vi "Maps Manager.vi"() -> ()   [LabVIEW 2014]
uses:
  <vilib>/Utility/miscctls.llb/LVPointDoubleTypeDef.ctl
  <vilib>/Utility/config.llb/Config Data RefNum.ctl
  Gps Map Graph enum.ctl
  Gps Map Graph config.ctl
  <vilib>/Utility/config.llb/Read Key (Double).vi
  <vilib>/Utility/config.llb/Write Key (Double).vi
  <vilib>/Utility/config.llb/Write Key (Path).vi
  <vilib>/ErrorRing/Error Ring.xnode
  <vilib>/Utility/config.llb/NI_LVConfig.lvlib
  My Graphs.lvlib
panel:
  in  "Points":T1[](array[typedef]) {"X" step=1e-05 format="%#_10g"; "Y" step=1e-05 format="%#_10g"}
  in  "Remove last":bool
  in  "Exit":bool
  out "Dati punto":string[][](array[string])
  in  "Save configurations":bool
  in  "North limit":dbl
  in  "South limit":dbl
  in  "East limit":dbl
  in  "West limit":dbl
  in  "Add point":bool
  in  "Load maps":bool
  in  "Load or create configurations":bool
  out "Zoom":cluster{"X":dbl, "Y":dbl}[](graph)
  out "My map":cluster{"X":dbl, "Y":dbl}[](graph)
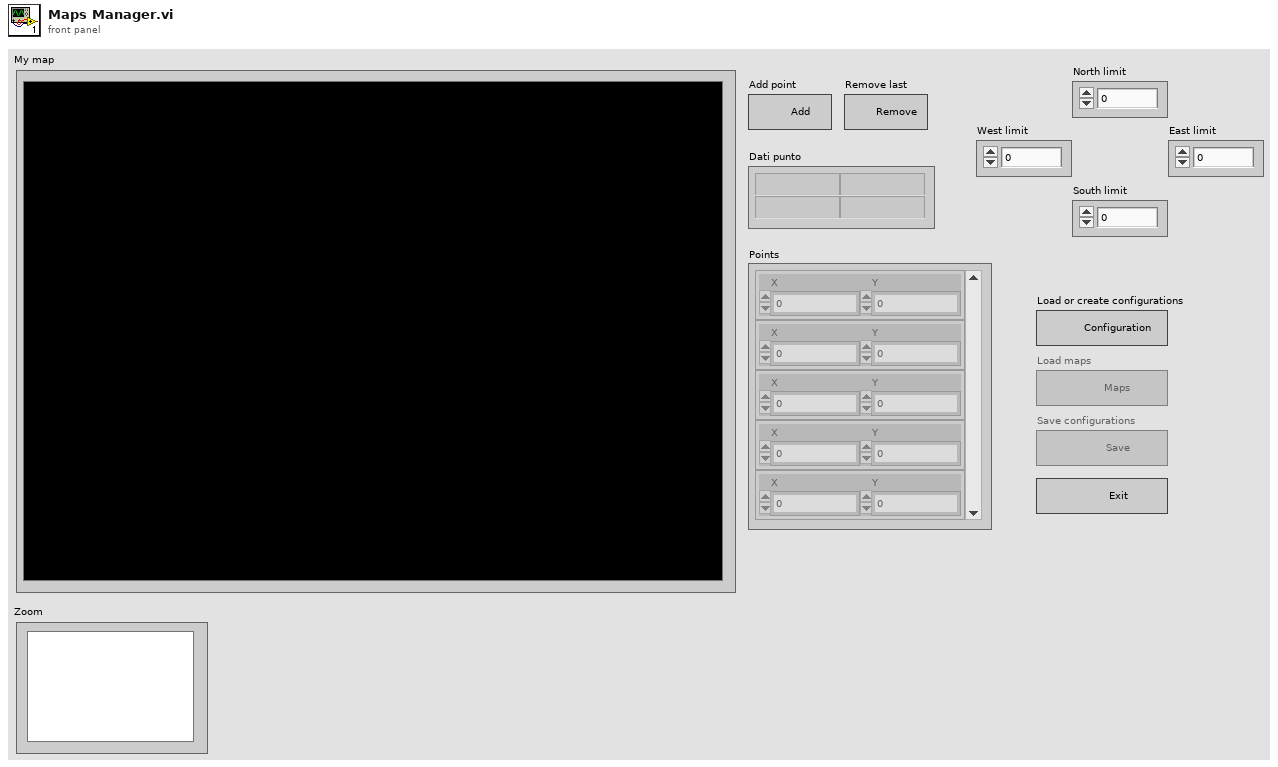
[diagram p1: front panel]
types:
  T1 = typedef "LVPointDoubleTypeDef.ctl" = cluster{"X":dbl, "Y":dbl}
  T2 = typedef "NI_LVConfig.lvlib/Config Data RefNum.ctl" = refnum<k1>
  T3 = cluster{"Config file?":bool, "Config file path":path, "Config file ref":T2, "Map files?":bool, "Big map file path":path, "Small map file path":path, "Path of points":T1[]}
  T4 = enum8{"Enabled", "Disabled", "Disabled and Grayed Out"}
  T5 = typedef "Gps Map Graph config.ctl" = cluster{"Config path":path, "Image path":path}
  T6 = typedef "My Graphs.lvlib/Gps Map Graph enum.ctl" = enum16{"Reset_ini", "Reset_txt", "SetValue"}
  T7 = typedef "imagedata.ctl" = cluster{"image type":i32, "image depth":i32, "image":u8[], "mask":u8[], "colors":u32[], "Rectangle":cluster{"left":i16, "top":i16, "right":i16, "bottom":i16}}
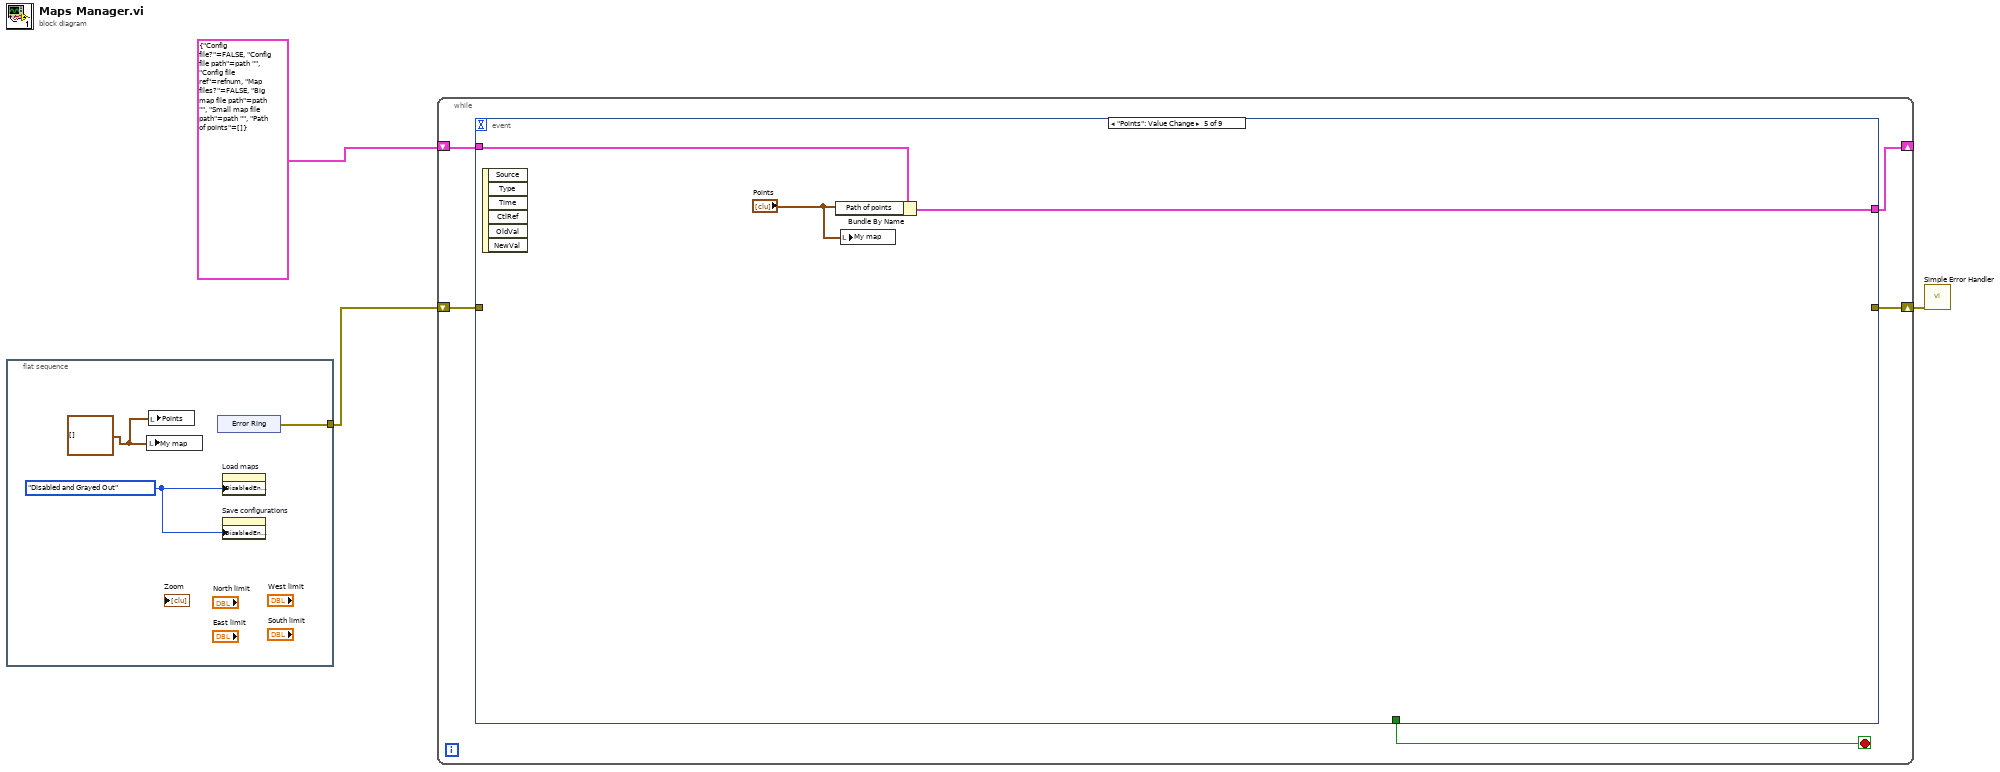
[diagram p0: block diagram]
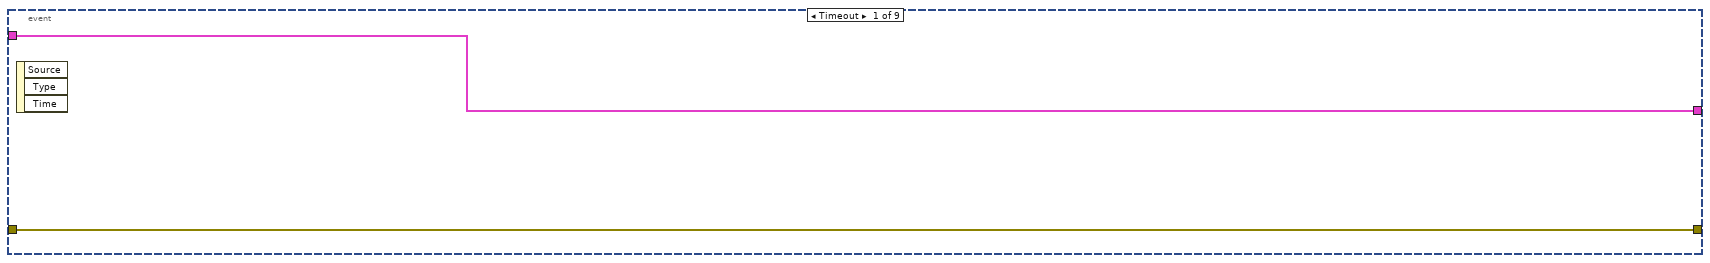
[diagram p2: hidden frame]
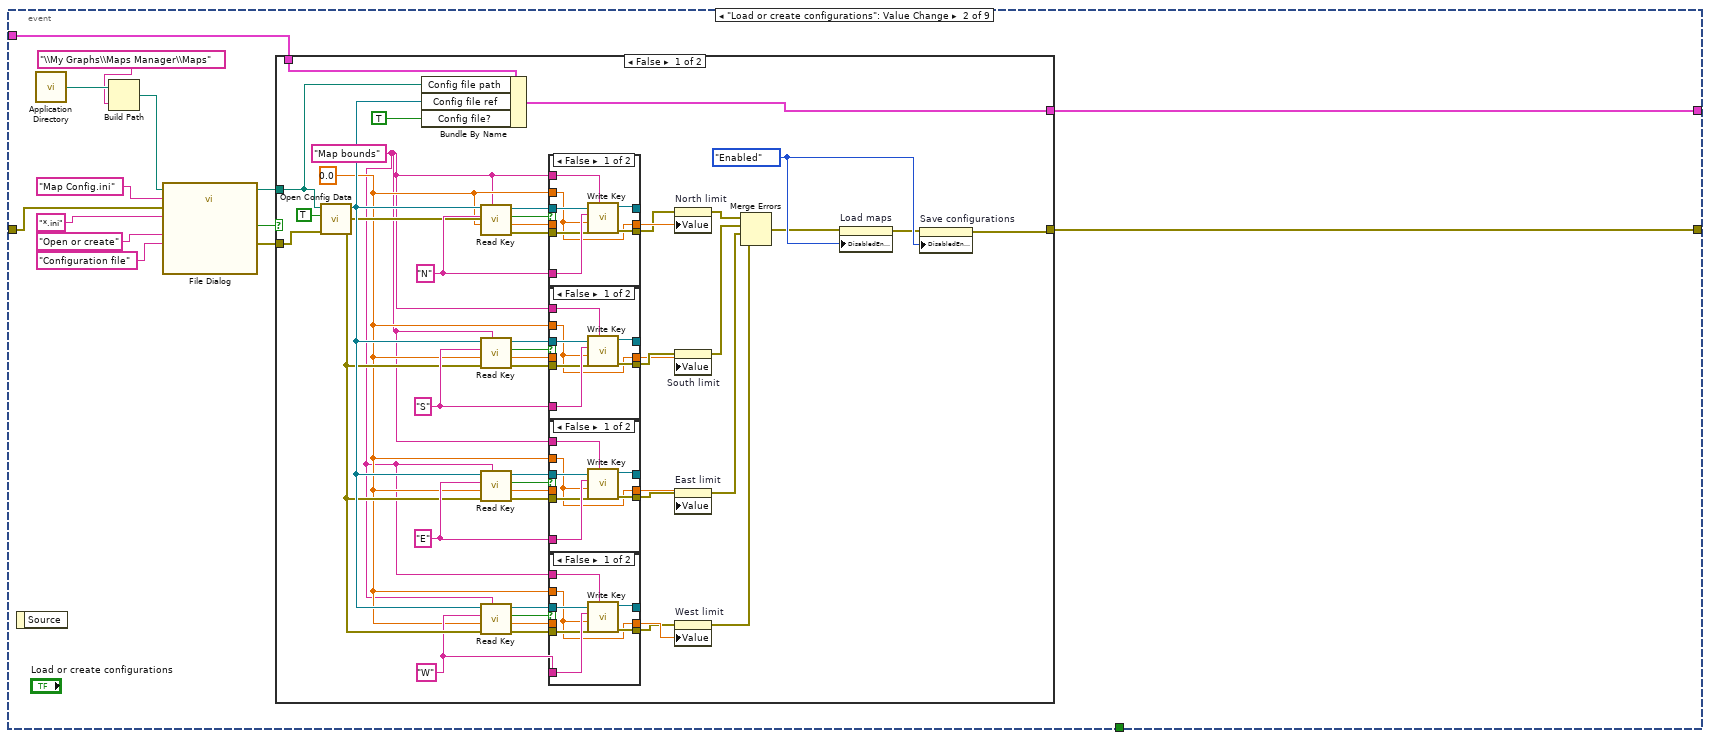
[diagram p3: hidden frame]
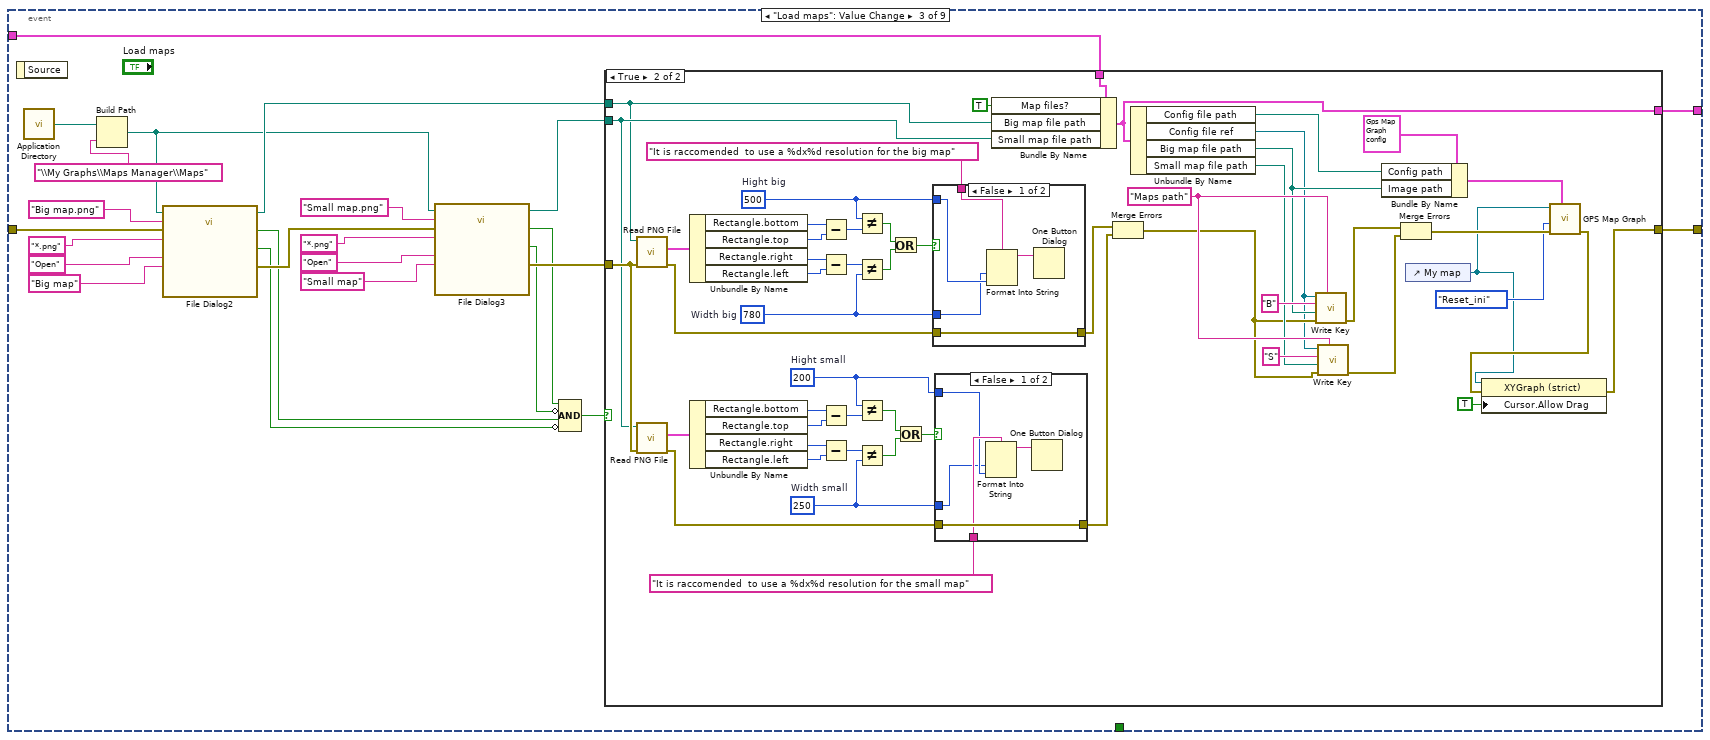
[diagram p9: hidden frame]
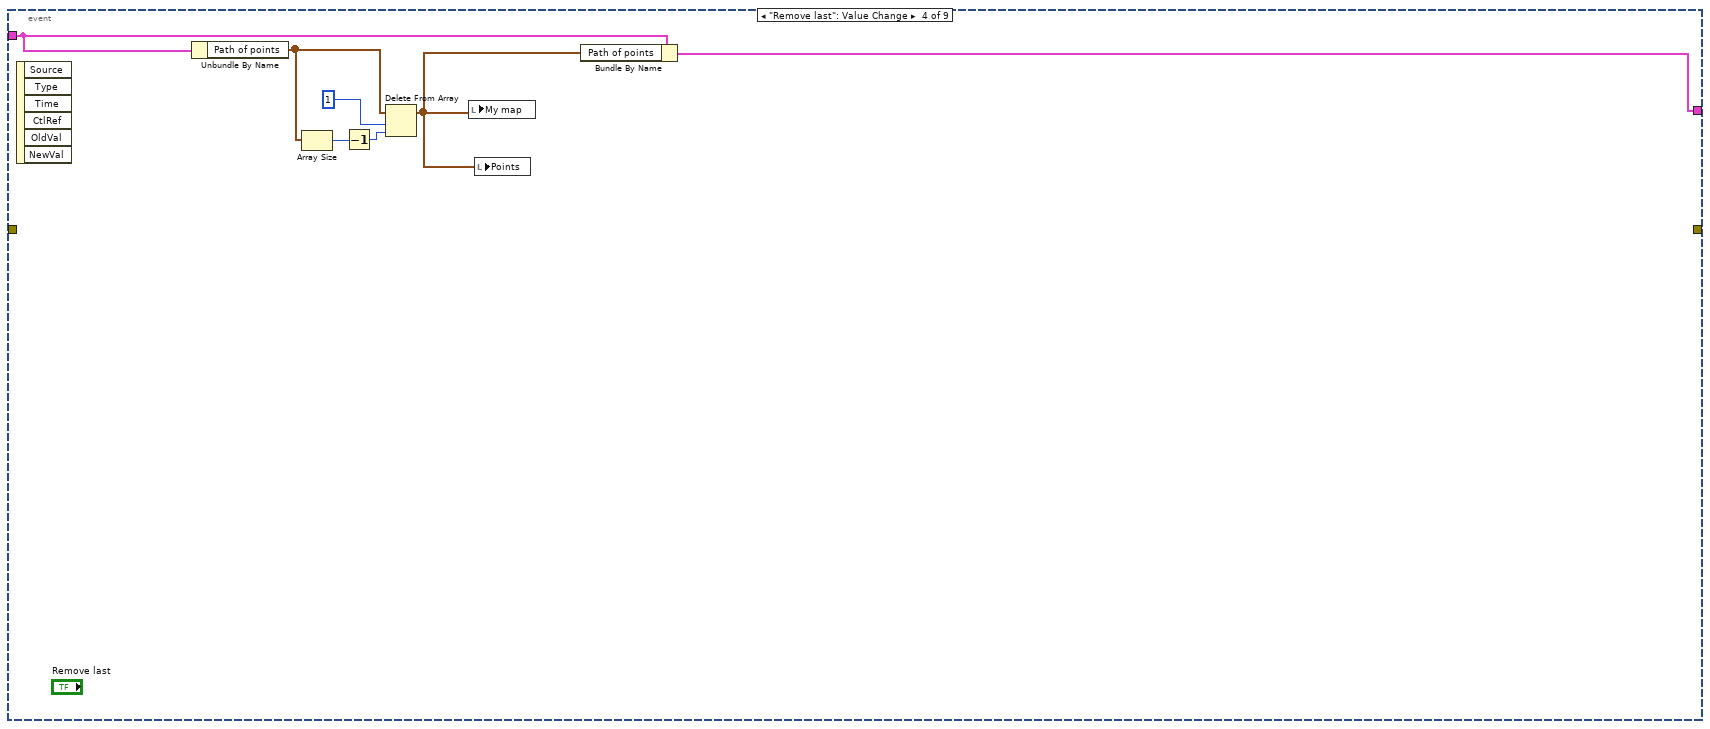
[diagram p13: hidden frame]
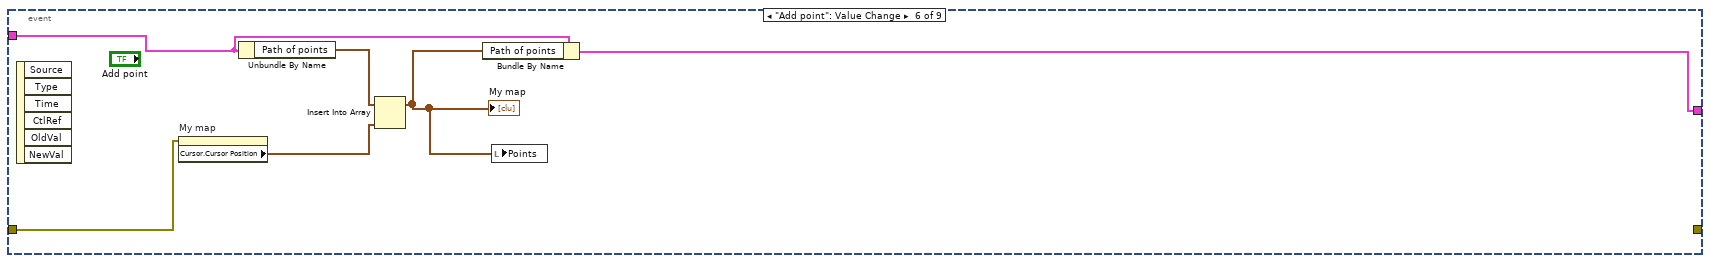
[diagram p14: hidden frame]
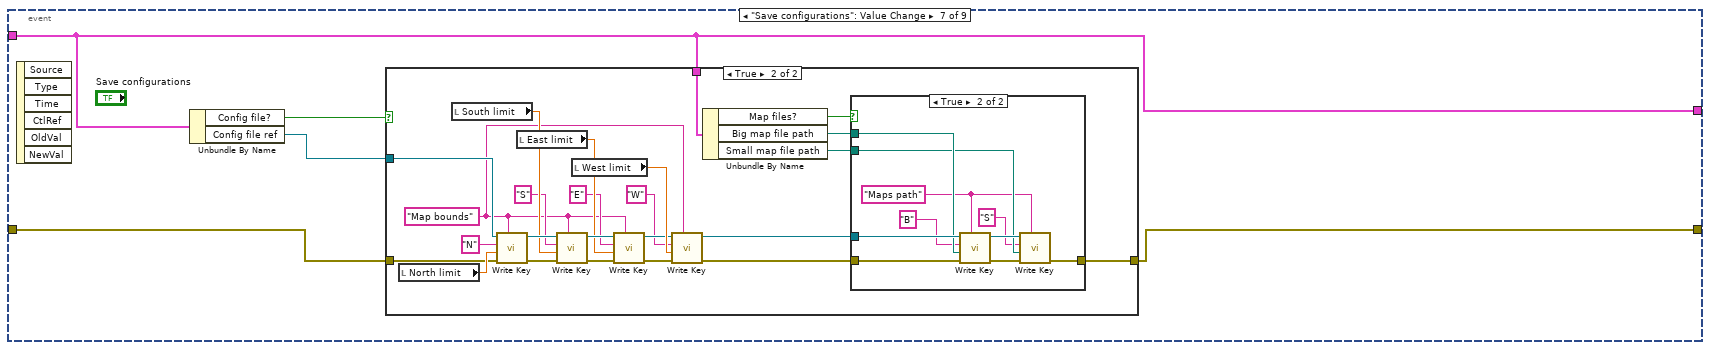
[diagram p15: hidden frame]
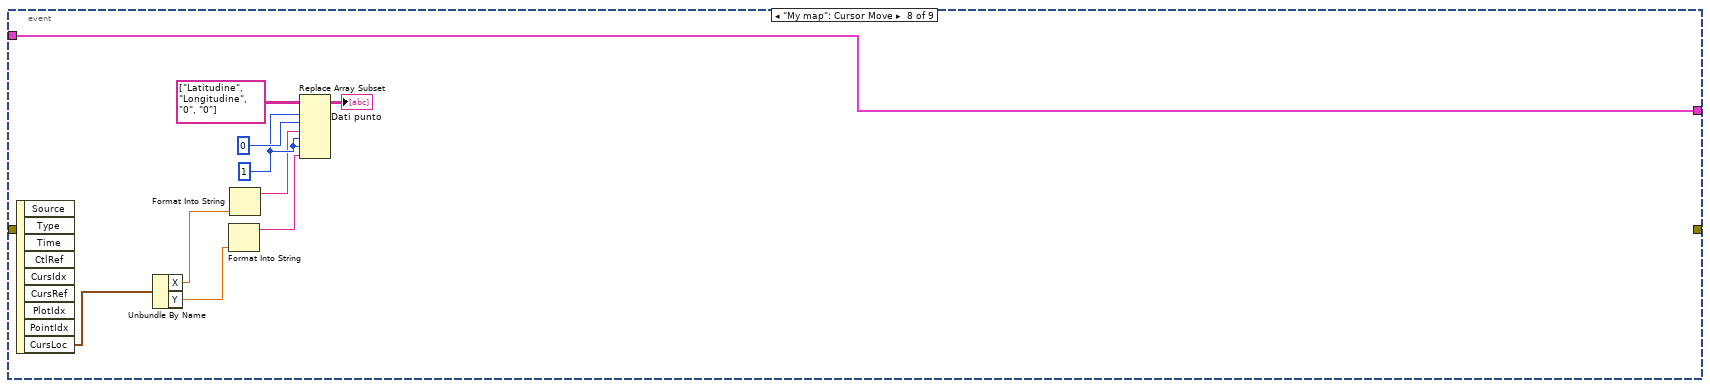
[diagram p18: hidden frame]
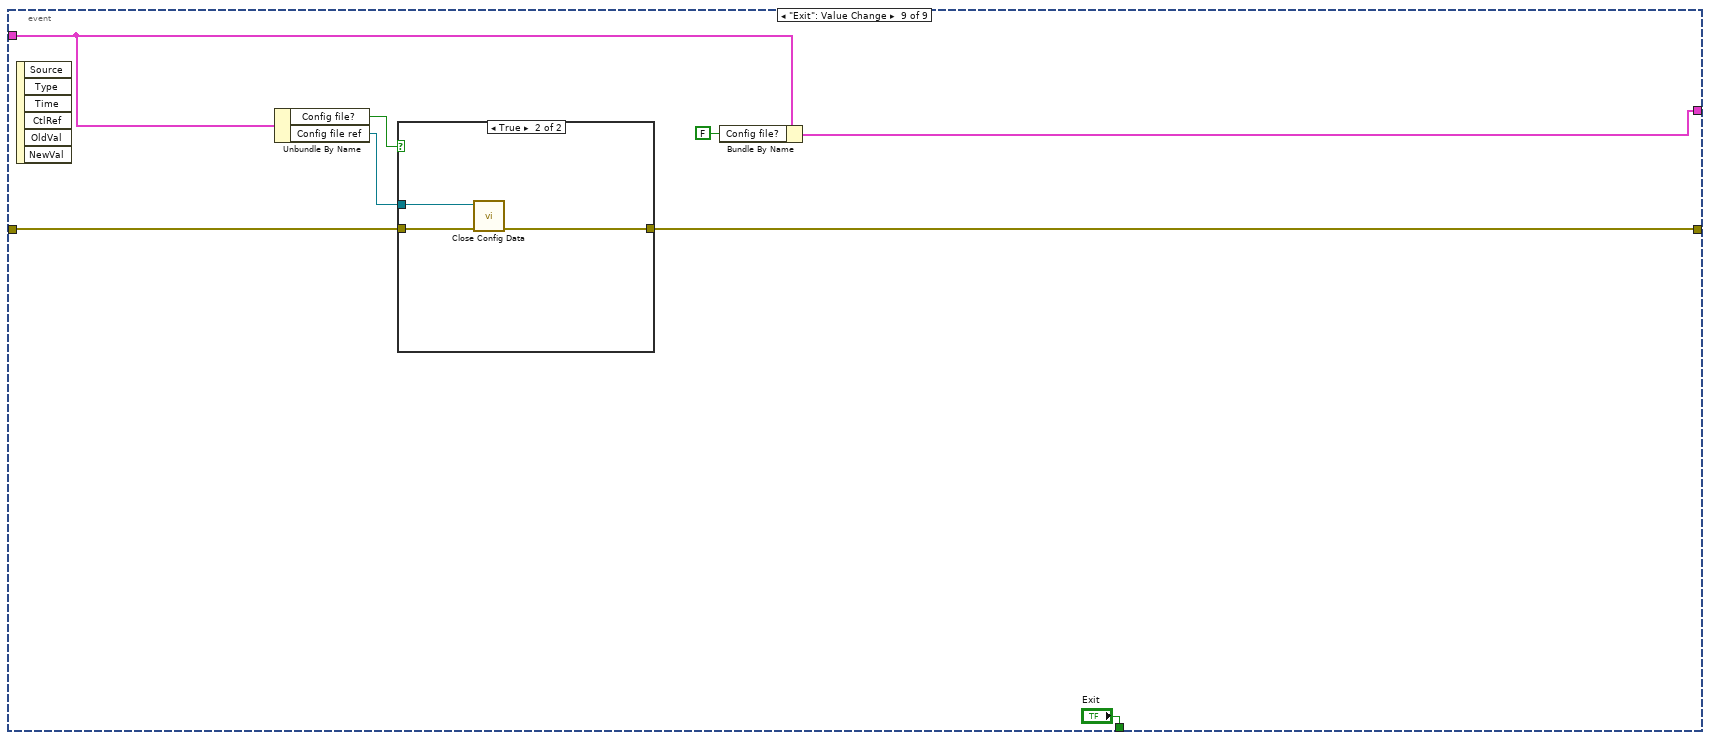
[diagram p19: hidden frame]
diagram:
  n1 = flat-sequence {
    tunnel: [w6] -> w3
    frame #0 {
      w4 = cluster{"X":i32, "Y":i32}[] [] ("My map")
      w5 = T4."Disabled and Grayed Out" ("Disabled")
      n2 = local write "My map"(w4) -> ()
      n3 = local write "Points"(w4) -> ()
      n4 = xnode "Error Ring"() -> ("error out"=w6:errorcluster)
      n5 = property on="Load maps" class="Bool"("DisabledEnum"=w5) -> ()  [unwired: 2 in, 2 out]
      n6 = property on="Save configurations" class="Bool"("DisabledEnum"=w5) -> ()  [unwired: 2 in, 2 out]
    }
  }
  n7 = while {
    shift-right: [w10] -> _
    shift-left: T3 {"Config file?"=FALSE, "Config file path"=path "", "Config file ref"=refnum, "Map files?"=FALSE, "Big map file path"=path "", "Small map file path"=path "", "Path of points"=[]} -> [w11]
    shift-right: [w9] -> w1
    shift-left: w3 -> [w12]
    stop <- w8 stop-if-true
    n8 = event shown="[4] \"Points\": Value Change" {
      selector: _ -> [_ _ _ _ _ _ _ _ _]
      dyn-events: _ -> [_ _ _ _ _ _ _ _ _]
      timeout: _ -> [_ _ _ _ _ _ _ _ _]
      tunnel: w12 -> [w13 w28 w136 _ _ w224 w227 _ w282]
      tunnel: [w13 w21 w120 _ _ _ w226 _ w281] -> w9
      tunnel: w11 -> [w14 w19 w121 w215 w218 w223 w225 w266 w278]
      tunnel: [w14 w18 w122 w214 w217 w222 w225 w266 w276] -> w10
      tunnel: [_ _ _ _ _ _ _ _ "Exit"] -> w8
      event Timeout {
        n9 = event-data() -> ()  [unwired: 1 in, 3 out]
      }
      event "Load or create configurations": Value Change {
        n10 = event-data() -> ()  [unwired: 1 in, 1 out]
        n11 = call <vilib>:"Application Directory.vi"() -> ("Application Directory"=w17:path)
        n12 = Build Path(base path=w17, name or relative path="\\My Graphs\\Maps Manager\\Maps") -> (appended path=w15:path)
        n13 = call "File Dialog"("start path"=w15, "prompt"="Configuration file", "button label"="Open or create", "default name"="Map Config.ini", "error in"=w28, "pattern (all files)"="*.ini") -> ("selected path"=w20:path, "cancelled"=w22:bool, "error out"=w23:errorcluster)  [unwired: 6 in, 1 out]
        n14 = case shown="False" w22 {
          tunnel: w23 -> [w71 w116]
          tunnel: [w30 w116] -> w21
          tunnel: w20 -> [w29 _]
          tunnel: w19 -> [w74 w115]
          tunnel: [w72 w115] -> w18
          frame False {
            w33 = T4."Enabled" ("Disabled")
            w46 = "W" ("key")
            w49 = "E" ("key")
            w48 = "S" ("key")
            w44 = "Map bounds" ("section")
            w65 = "N" ("key")
            w45 = 0.0 ("default value")
            n15 = call <vilib>:"Open Config Data.vi"("error in (no error)"=w71, "create file if necessary (T)"=TRUE, "configuration file path"=w29) -> ("error out"=w47:errorcluster, "refnum"=w50:T2)  [unwired: 6 in, 1 out]
            n16 = Bundle By Name(cluster=w74, "Config file path"=w29, "Config file ref"=w50, "Config file?"=TRUE) -> (w72:T3)
            n17 = call-poly <vilib>:"Read Key.vi"("section"=w44, "error in (no error)"=w47, "default value"=w45, "key"=w65, "refnum"=w50) -> ("error out"=w66:errorcluster, "value"=w67:dbl, "found?"=w69:bool, "refnum out"=w68:T2)  [unwired: 3 in]
            n18 = call-poly <vilib>:"Read Key.vi"("section"=w44, "error in (no error)"=w47, "default value"=w45, "key"=w48, "refnum"=w50) -> ("error out"=w59:errorcluster, "value"=w60:dbl, "found?"=w62:bool, "refnum out"=w61:T2)  [unwired: 3 in]
            n19 = call-poly <vilib>:"Read Key.vi"("section"=w44, "error in (no error)"=w47, "default value"=w45, "key"=w49, "refnum"=w50) -> ("error out"=w55:errorcluster, "value"=w56:dbl, "found?"=w58:bool, "refnum out"=w57:T2)  [unwired: 3 in]
            n20 = call-poly <vilib>:"Read Key.vi"("section"=w44, "error in (no error)"=w47, "default value"=w45, "key"=w46, "refnum"=w50) -> ("error out"=w51:errorcluster, "value"=w52:dbl, "found?"=w54:bool, "refnum out"=w53:T2)  [unwired: 3 in]
            n21 = case shown="False" w69 {
              tunnel: w68 -> [w111 w112]
              tunnel: w67 -> [_ w113]
              tunnel: w66 -> [w108 w114]
              tunnel: w65 -> [w109 _]
              tunnel: w44 -> [w110 _]
              tunnel: w45 -> [w106 _]
              tunnel: [w107 w114] -> w63
              tunnel: [w106 w113] -> w64
              tunnel: [w105 w112] -> _
              frame False {
                n22 = call-poly <vilib>:"Write Key.vi"("section"=w110, "error in (no error)"=w108, "value"=w106, "key"=w109, "refnum"=w111) -> ("error out"=w107:errorcluster, "refnum out"=w105:T2)  [unwired: 4 in, 1 out]
              }
              frame True {
              }
            }
            n23 = case shown="False" w62 {
              tunnel: w61 -> [w101 w102]
              tunnel: w60 -> [_ w103]
              tunnel: w59 -> [w98 w104]
              tunnel: w48 -> [w99 _]
              tunnel: w44 -> [w100 _]
              tunnel: w45 -> [w96 _]
              tunnel: [w97 w104] -> w43
              tunnel: [w96 w103] -> w38
              tunnel: [w95 w102] -> _
              frame False {
                n24 = call-poly <vilib>:"Write Key.vi"("section"=w100, "error in (no error)"=w98, "value"=w96, "key"=w99, "refnum"=w101) -> ("error out"=w97:errorcluster, "refnum out"=w95:T2)  [unwired: 4 in, 1 out]
              }
              frame True {
              }
            }
            n25 = case shown="False" w58 {
              tunnel: w57 -> [w91 w92]
              tunnel: w56 -> [_ w93]
              tunnel: w55 -> [w88 w94]
              tunnel: w49 -> [w89 _]
              tunnel: w44 -> [w90 _]
              tunnel: w45 -> [w86 _]
              tunnel: [w87 w94] -> w39
              tunnel: [w86 w93] -> w40
              tunnel: [w85 w92] -> _
              frame False {
                n26 = call-poly <vilib>:"Write Key.vi"("section"=w90, "error in (no error)"=w88, "value"=w86, "key"=w89, "refnum"=w91) -> ("error out"=w87:errorcluster, "refnum out"=w85:T2)  [unwired: 4 in, 1 out]
              }
              frame True {
              }
            }
            n27 = case shown="False" w54 {
              tunnel: w53 -> [w81 w82]
              tunnel: w52 -> [_ w83]
              tunnel: w51 -> [w78 w84]
              tunnel: w46 -> [w79 _]
              tunnel: w44 -> [w80 _]
              tunnel: w45 -> [w76 _]
              tunnel: [w77 w84] -> w41
              tunnel: [w76 w83] -> w42
              tunnel: [w75 w82] -> _
              frame False {
                n28 = call-poly <vilib>:"Write Key.vi"("section"=w80, "error in (no error)"=w78, "value"=w76, "key"=w79, "refnum"=w81) -> ("error out"=w77:errorcluster, "refnum out"=w75:T2)  [unwired: 4 in, 1 out]
              }
              frame True {
              }
            }
            n29 = property on="North limit" class="DigNum (strict)"(error in=w63, "Value"=w64) -> (error out=w37:errorcluster)  [unwired: 1 in, 1 out]
            n30 = property on="South limit" class="DigNum (strict)"(error in=w43, "Value"=w38) -> (error out=w36:errorcluster)  [unwired: 1 in, 1 out]
            n31 = property on="East limit" class="DigNum (strict)"(error in=w39, "Value"=w40) -> (error out=w35:errorcluster)  [unwired: 1 in, 1 out]
            n32 = property on="West limit" class="DigNum (strict)"(error in=w41, "Value"=w42) -> (error out=w34:errorcluster)  [unwired: 1 in, 1 out]
            n33 = Merge Errors(w37, w36, w35, w34) -> (w32:errorcluster)
            n34 = property on="Load maps" class="Bool"(error in=w32, "DisabledEnum"=w33) -> (error out=w31:errorcluster)  [unwired: 1 in, 1 out]
            n35 = property on="Save configurations" class="Bool"(error in=w31, "DisabledEnum"=w33) -> (error out=w30:errorcluster)  [unwired: 1 in, 1 out]
          }
          frame True {
          }
        }
      }
      event "Load maps": Value Change {
        n36 = event-data() -> ()  [unwired: 1 in, 1 out]
        n37 = call <vilib>:"Application Directory.vi"() -> ("Application Directory"=w119:path)
        n38 = Build Path(base path=w119, name or relative path="\\My Graphs\\Maps Manager\\Maps") -> (appended path=w118:path)
        n39 = call "File Dialog2"("start path"=w118, "prompt"="Big map", "button label"="Open", "default name"="Big map.png", "error in"=w136, "pattern (all files)"="*.png") -> ("selected path"=w124:path, "exists"=w127:bool, "cancelled"=w126:bool, "error out"=w131:errorcluster)  [unwired: 6 in]
        n40 = call "File Dialog3"("start path"=w118, "prompt"="Small map", "button label"="Open", "default name"="Small map.png", "error in"=w131, "pattern (all files)"="*.png") -> ("selected path"=w123:path, "exists"=w129:bool, "cancelled"=w128:bool, "error out"=w130:errorcluster)  [unwired: 6 in]
        n41 = Compound Arithmetic op=AND(w129, invert w128, w127, invert w126) -> (w125:bool)
        n42 = case shown="True" w125 {
          tunnel: w130 -> [w142 w186]
          tunnel: [w142 w145] -> w120
          tunnel: w124 -> [_ w160]
          tunnel: w123 -> [_ w164]
          tunnel: [w141 w162] -> w122
          tunnel: w121 -> [w141 w163]
          frame False {
          }
          frame True {
            w158 = "Maps path" ("section")
            w170 = i16 780  # Width big
            w171 = i16 500  # Hight big
            w168 = i16 250  # Width small
            w169 = i16 200  # Hight small
            n43 = call <vilib>:"Read PNG File.vi"("error in (no error)"=w186, "path to PNG file"=w160) -> ("error out"=w174:errorcluster, "image data"=w196:T7)  [unwired: 7 in, 1 out]
            n44 = call <vilib>:"Read PNG File.vi"("error in (no error)"=w186, "path to PNG file"=w164) -> ("error out"=w175:errorcluster, "image data"=w191:T7)  [unwired: 7 in, 1 out]
            n45 = Unbundle By Name(w196) -> ("Rectangle.bottom"=w192:i16, "Rectangle.top"=w193:i16, "Rectangle.right"=w195:i16, "Rectangle.left"=w194:i16)
            n46 = Unbundle By Name(w191) -> ("Rectangle.bottom"=w187:i16, "Rectangle.top"=w188:i16, "Rectangle.right"=w190:i16, "Rectangle.left"=w189:i16)
            n47 = Subtract(x=w192, y=w193) -> (x-y=w185:i16)
            n48 = Subtract(x=w195, y=w194) -> (x-y=w184:i16)
            n49 = Subtract(x=w187, y=w188) -> (x-y=w183:i16)
            n50 = Subtract(x=w190, y=w189) -> (x-y=w182:i16)
            n51 = Not Equal?(x=w171, y=w185) -> (x != y?=w181:bool)
            n52 = Not Equal?(x=w184, y=w170) -> (x != y?=w180:bool)
            n53 = Not Equal?(x=w169, y=w183) -> (x != y?=w179:bool)
            n54 = Not Equal?(x=w182, y=w168) -> (x != y?=w178:bool)
            n55 = Or(x=w181, y=w180) -> (x .or. y?=w176:bool)
            n56 = Or(x=w179, y=w178) -> (x .or. y?=w177:bool)
            n57 = case shown="False" w176 {
              tunnel: w174 -> [w201 w202]
              tunnel: [w201 w202] -> w173
              tunnel: w171 -> [w198 _]
              tunnel: w170 -> [w197 _]
              tunnel: "It is raccomended  to use a %dx%d resolution for the big map" -> [w199 _]
              frame False {
                n58 = Format Into String(format string=w199, w197, w198) -> (resulting string=w200:string)  [unwired: 2 in, 1 out]
                n59 = One Button Dialog(message=w200) -> ()  [unwired: 1 in, 1 out]
              }
              frame True {
              }
            }
            n60 = case shown="False" w177 {
              tunnel: w175 -> [w207 w208]
              tunnel: [w207 w208] -> w172
              tunnel: w169 -> [w204 _]
              tunnel: w168 -> [w203 _]
              tunnel: "It is raccomended  to use a %dx%d resolution for the small map" -> [w205 _]
              frame False {
                n61 = Format Into String(format string=w205, w203, w204) -> (resulting string=w206:string)  [unwired: 2 in, 1 out]
                n62 = One Button Dialog(message=w206) -> ()  [unwired: 1 in, 1 out]
              }
              frame True {
              }
            }
            n63 = Bundle By Name(cluster=w163, "Map files?"=TRUE, "Big map file path"=w160, "Small map file path"=w164) -> (w162:T3)
            n64 = Merge Errors(w173, w172) -> (w156:errorcluster)
            n65 = Unbundle By Name(w162) -> ("Config file path"=w148:path, "Config file ref"=w147:T2, "Big map file path"=w149:path, "Small map file path"=w157:path)
            n66 = call-poly <vilib>:"Write Key.vi"("section"=w158, "error in (no error)"=w156, "value"=w149, "key"="B", "refnum"=w147) -> ("error out"=w154:errorcluster)  [unwired: 4 in, 2 out]
            n67 = call-poly <vilib>:"Write Key.vi"("section"=w158, "error in (no error)"=w156, "value"=w157, "key"="S", "refnum"=w147) -> ("error out"=w155:errorcluster)  [unwired: 4 in, 2 out]
            n68 = Bundle By Name(cluster=T5 {"Config path"=path "E:/Dropbox/Condivise/Condivisa con Fausto Petruzzelli/Test/GPS/Test_gps_3/mappa1.txt", "Image path"=path "E:/Dropbox/Condivise/Condivisa con Fausto Petruzzelli/Test/GPS/Test_gps_3/mappa1.png"} ("Map config"), "Config path"=w148, "Image path"=w149) -> (w151:T5)
            n69 = Merge Errors(w154, w155) -> (w153:errorcluster)
            n70 = control-ref of="My map"() -> (w144:refnum<vi>)
            n71 = call "GPS Map Graph.vi"("Map config"=w151, "Error In"=w153, "Function"=Gps_Map_Graph_enum."Reset_ini", "Map ref in"=w144) -> ("Error Out"=w146:errorcluster)  [unwired: 6 in, 1 out]
            n72 = property on="Property Node" class="XYGraph (strict)"(reference=w144, error in=w146, "Cursor.Allow Drag"=TRUE) -> (error out=w145:errorcluster)  [unwired: 1 out]
          }
        }
      }
      event "Remove last": Value Change {
        n73 = event-data() -> ()  [unwired: 1 in, 6 out]
        n74 = Unbundle By Name(w215) -> ("Path of points"=w212:T1[])
        n75 = Array Size(array=w212) -> (size(s)=w211:i32)
        n76 = Decrement(x=w211) -> (x-1=w210:i32)
        n77 = Delete From Array(array=w212, length=1, index=w210) -> (array with subset deleted=w209:T1[])  [unwired: 1 out]
        n78 = local write "My map"(w209) -> ()
        n79 = local write "Points"(w209) -> ()
        n80 = Bundle By Name(cluster=w215, "Path of points"=w209) -> (w214:T3)
      }
      event "Points": Value Change {
        n81 = event-data() -> ()  [unwired: 1 in, 6 out]
        n82 = Bundle By Name(cluster=w218, "Path of points"="Points") -> (w217:T3)
        n83 = local write "My map"("Points") -> ()
      }
      event "Add point": Value Change {
        n84 = event-data() -> ()  [unwired: 1 in, 6 out]
        n85 = property on="My map" class="XYGraph (strict)"(error in=w224) -> ("Cursor.Cursor Position"=w220:T1)  [unwired: 1 in, 2 out]
        n86 = Unbundle By Name(w223) -> ("Path of points"=w221:T1[])
        n87 = Insert Into Array(array=w221, new element=w220) -> (w219:T1[])  [unwired: 1 in]
        "My map" <- w219
        n88 = Bundle By Name(cluster=w223, "Path of points"=w219) -> (w222:T3)
        n89 = local write "Points"(w219) -> ()
      }
      event "Save configurations": Value Change {
        n90 = event-data() -> ()  [unwired: 1 in, 6 out]
        n91 = Unbundle By Name(w225) -> ("Config file?"=w228:bool, "Config file ref"=w229:T2)
        n92 = case shown="True" w228 {
          tunnel: w229 -> [_ w254]
          tunnel: w227 -> [w230 w251]
          tunnel: w225 -> [_ w237]
          tunnel: [w230 w231] -> w226
          frame False {
          }
          frame True {
            w238 = "Map bounds" ("section")
            n93 = local read "North limit"() -> (w252:dbl)
            n94 = local read "South limit"() -> (w243:dbl)
            n95 = call-poly <vilib>:"Write Key.vi"("section"=w238, "error in (no error)"=w251, "value"=w252, "key"="N", "refnum"=w254) -> ("error out"=w247:errorcluster, "refnum out"=w246:T2)  [unwired: 4 in, 1 out]
            n96 = local read "East limit"() -> (w242:dbl)
            n97 = call-poly <vilib>:"Write Key.vi"("section"=w238, "error in (no error)"=w247, "value"=w243, "key"="S", "refnum"=w246) -> ("error out"=w248:errorcluster, "refnum out"=w245:T2)  [unwired: 4 in, 1 out]
            n98 = local read "West limit"() -> (w250:dbl)
            n99 = call-poly <vilib>:"Write Key.vi"("section"=w238, "error in (no error)"=w248, "value"=w242, "key"="E", "refnum"=w245) -> ("error out"=w249:errorcluster, "refnum out"=w244:T2)  [unwired: 4 in, 1 out]
            n100 = call-poly <vilib>:"Write Key.vi"("section"=w238, "error in (no error)"=w249, "value"=w250, "key"="W", "refnum"=w244) -> ("error out"=w235:errorcluster, "refnum out"=w234:T2)  [unwired: 4 in, 1 out]
            n101 = Unbundle By Name(w237) -> ("Map files?"=w236:bool, "Big map file path"=w233:path, "Small map file path"=w232:path)
            n102 = case shown="True" w236 {
              tunnel: w235 -> [w255 w264]
              tunnel: w234 -> [_ w263]
              tunnel: w233 -> [_ w261]
              tunnel: w232 -> [_ w260]
              tunnel: [w255 w256] -> w231
              frame False {
              }
              frame True {
                w259 = "Maps path" ("section")
                n103 = call-poly <vilib>:"Write Key.vi"("section"=w259, "error in (no error)"=w264, "value"=w261, "key"="B", "refnum"=w263) -> ("error out"=w265:errorcluster, "refnum out"=w262:T2)  [unwired: 4 in, 1 out]
                n104 = call-poly <vilib>:"Write Key.vi"("section"=w259, "error in (no error)"=w265, "value"=w260, "key"="S", "refnum"=w262) -> ("error out"=w256:errorcluster)  [unwired: 4 in, 2 out]
              }
            }
          }
        }
      }
      event "My map": Cursor Move {
        w271 = 1 ("index (row)")
        n105 = event-data() -> ("CursLoc"=w275:cluster{"X":dbl, "Y":dbl})  [unwired: 1 in, 8 out]
        n106 = Unbundle By Name(w275) -> ("X"=w270:dbl, "Y"=w267:dbl)
        n107 = Format Into String(w267) -> (resulting string=w268:string)  [unwired: 3 in, 1 out]
        n108 = Format Into String(w270) -> (resulting string=w269:string)  [unwired: 3 in, 1 out]
        n109 = Replace Array Subset(array=string[][] [["Latitudine", "Longitudine"], ["0", "0"]], new element #1=w269, index (row) #1=w271, index (col) #1=0 ("disabled index (col)"), new element #2=w268, index (row) #2=w271, index (col) #2=w271) -> (→"Dati punto":string[][])
      }
      event "Exit": Value Change {
        n110 = event-data() -> ()  [unwired: 1 in, 6 out]
        n111 = Unbundle By Name(w278) -> ("Config file?"=w279:bool, "Config file ref"=w280:T2)
        n112 = case shown="True" w279 {
          tunnel: w282 -> [w284 w287]
          tunnel: w280 -> [_ w286]
          tunnel: [w284 w285] -> w281
          frame False {
          }
          frame True {
            n113 = call <vilib>:"Close Config Data.vi"("error in (no error)"=w287, "refnum"=w286) -> ("error out"=w285:errorcluster)  [unwired: 8 in, 1 out]
          }
        }
        n114 = Bundle By Name(cluster=w278, "Config file?"=FALSE) -> (w276:T3)
      }
    }
  }
  n115 = call <vilib>:"Simple Error Handler.vi"("error in (no error)"=w1) -> ()  [unwired: 4 in, 5 out]
